vi "Install Package via Custom System Exec.vi"(8 "error in":errorcluster, 9 "include recommended packages? (F)":bool, 10 "version":string, 11 "package name":string) -> (0 "error out":errorcluster, 2 "installed version":string, 3 "package name out":string)   [LabVIEW 2019]
doc: "Installs the specified package on this computer.\n\nNote: This VI will launch a Windows dialog asking for permission to run and requires the user to have admin rights.\n\nINPUT(s)\n<B>Package name</B>: Specifies the package to install.\n\n<B>Version</B>:\nIf the version input is left unwired and no version of the package is currently installed, this VI will install the latest version of the package available from the registered feeds on the computer.\nIf the version input is left unwired and any version of the package is currently installed, this VI will output an error.\n\nIf the version input is wired and a different version of the package is installed, this VI will upgrade or downgrade the package to the specified version.\nIf the version input is wired and the specified version of the package is already installed, this VI will output an error.\n\n<B>Include recommended packages</B>: Also install all recommended packages of the specified package.\n\nOUTPUT(s)\n<B>Package name</B>: Outputs the requested package to install.\n\n<B>Installed version</B>: Outputs the currently installed version of the specified package after this VI tries to install the package.\n\nNIPM API 3.2.1.9\nNational Instruments\nCopyright (c) 2020, National Instruments"
uses:
  <vilib>/National Instruments/NIPM API (Beta)/NIPM_API.lvlib
  <vilib>/National Instruments/NIPM API (Beta)/_support/Version Comparison Operator.ctl
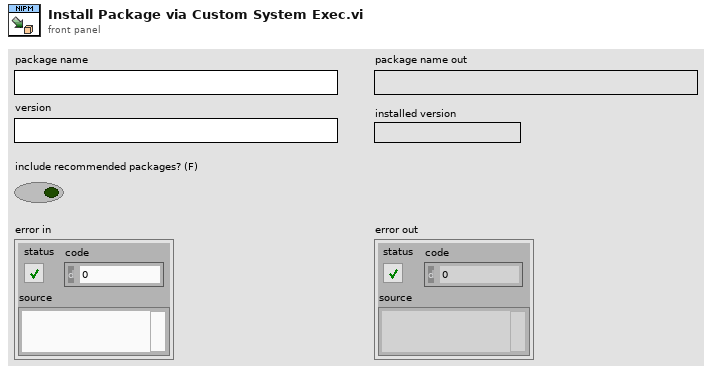
[diagram p1: front panel]
types:
  T1 = typedef "NIPM_API.lvlib/Version Comparison Operator.ctl" = enum16{">", ">=", "=", "!=", "<=", "<"}
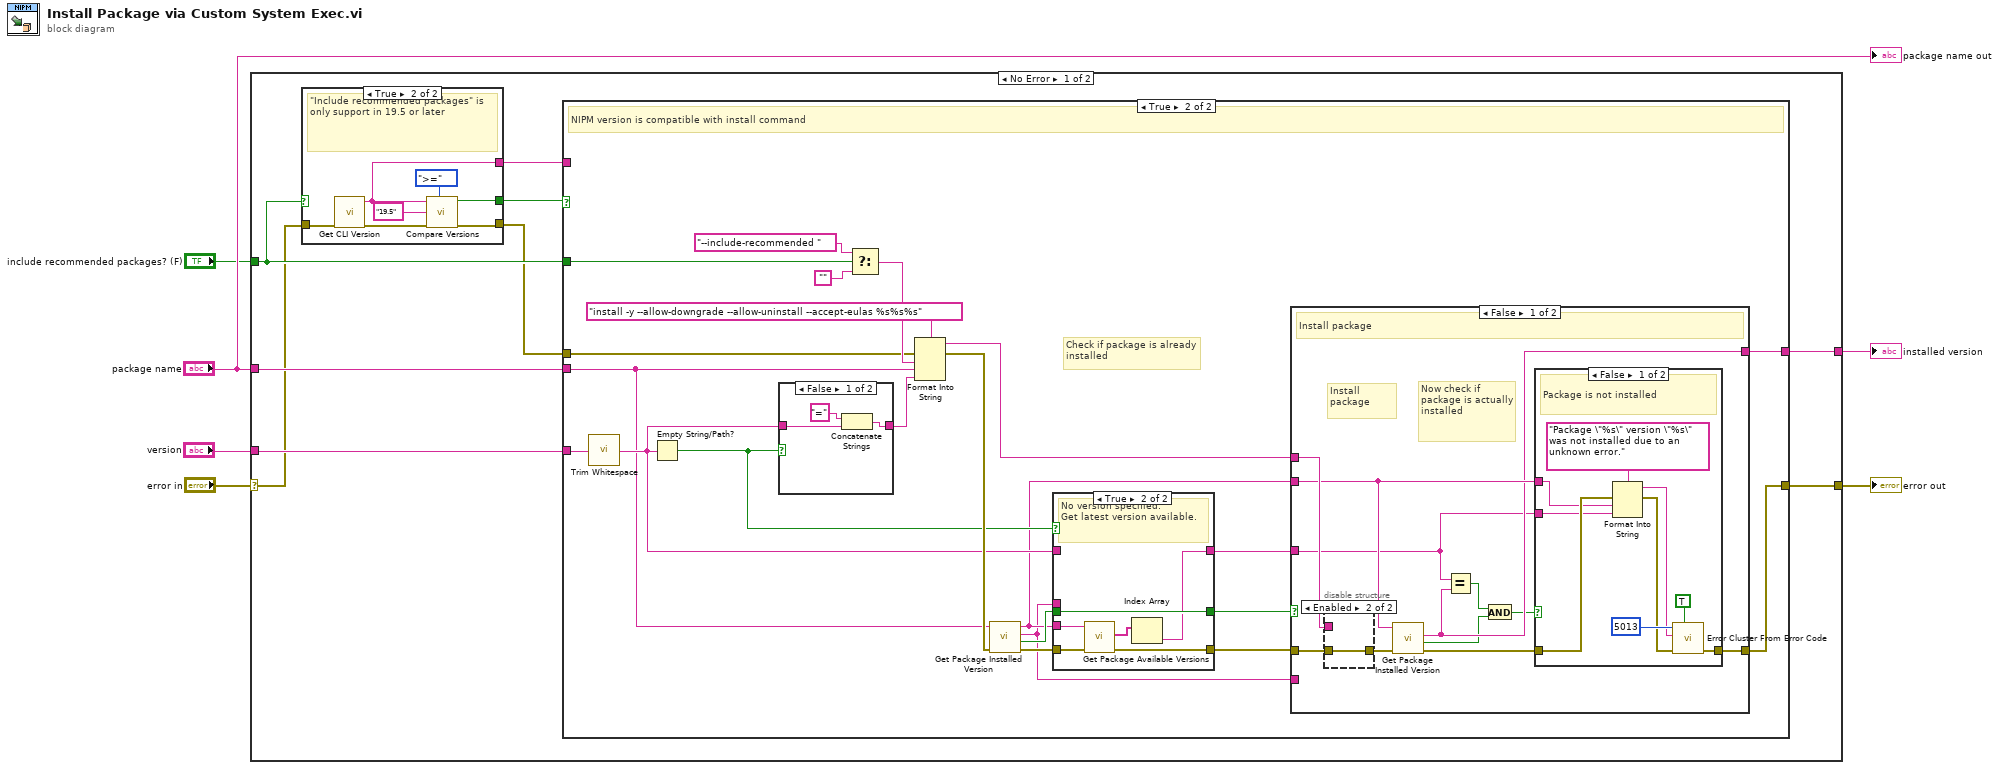
[diagram p0: block diagram]
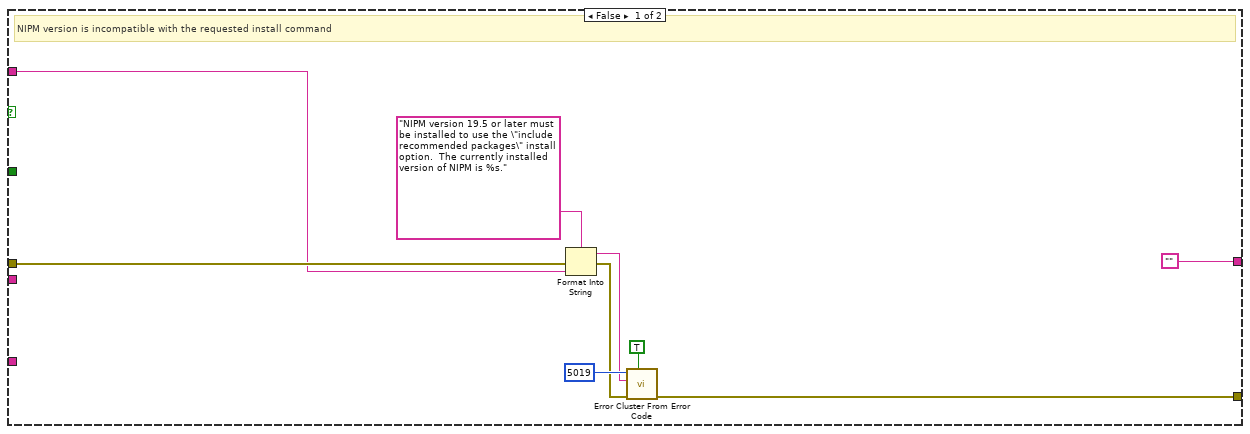
[diagram p2: hidden frame]
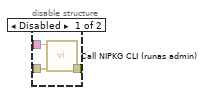
[diagram p3: hidden frame]
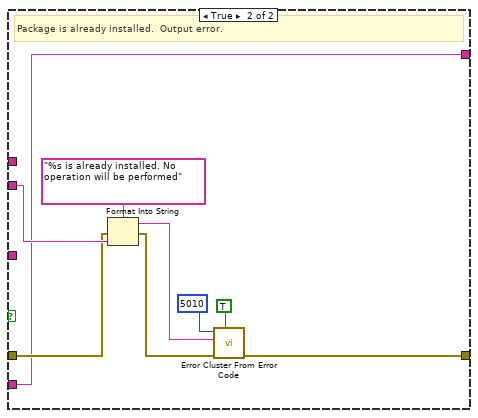
[diagram p5: hidden frame]
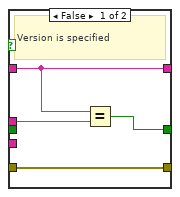
[diagram p6: hidden frame]
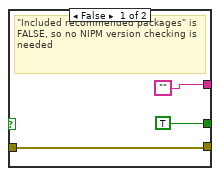
[diagram p8: hidden frame]
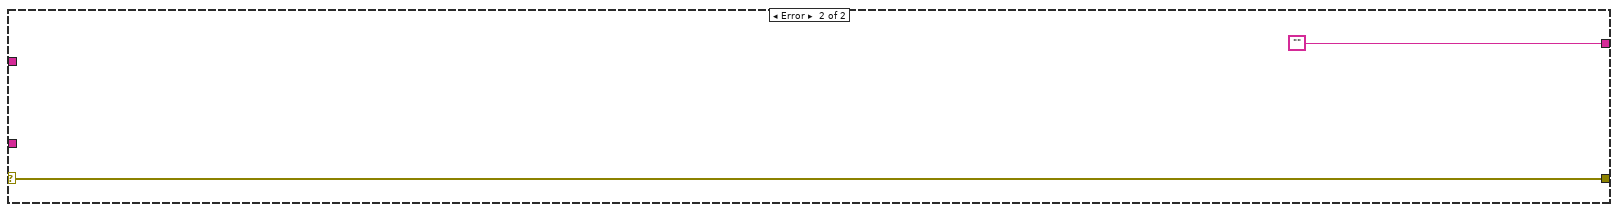
[diagram p9: hidden frame]
diagram:
  n1 = case shown="No Error" "error in" {
    selector: "error in" -> [w10 w106]
    tunnel: [w15 w106] -> w5
    tunnel: "package name" -> [w12 _]
    tunnel: "version" -> [w14 _]
    tunnel: [w13 "" ("standard output")] -> w2
    tunnel: "include recommended packages? (F)" -> [w11 _]
    frame No Error {
      n2 = case shown="True" w11 {
        tunnel: w10 -> [w97 w101]
        tunnel: [w97 w100] -> w9
        tunnel: [TRUE ("Satisfied?") w99] -> w8
        tunnel: ["" w98] -> w7
        frame False {
          # "\"Included recommended packages\" is FALSE, so no NIPM version checking is needed"
        }
        frame True {
          # "\"Include recommended packages\" is only support in 19.5 or later"
          n3 = call <vilib>:"Get CLI Version.vi"("error in"=w101) -> ("error out"=w102:errorcluster, "full version string"=w98:string)  [unwired: 9 in]
          n4 = call <vilib>:"Compare Versions.vi"("operator"=Version_Comparison_Operator.">=", "error in"=w102, "version y"="19.5", "version x"=w98) -> ("error out"=w100:errorcluster, "Satisfied?"=w99:bool)  [unwired: 6 in]
        }
      }
      n5 = case shown="True" w8 {
        tunnel: [w18 w42] -> w15
        tunnel: w14 -> [_ w40]
        tunnel: ["" w38] -> w13
        tunnel: w12 -> [_ w28]
        tunnel: w11 -> [_ w26]
        tunnel: w9 -> [w19 w25]
        tunnel: w7 -> [w16 _]
        frame False {
          # "NIPM version is incompatible with the requested install command"
          n6 = Format Into String(format string="NIPM version 19.5 or later must be installed to use the \"include recommended packages\" install option.  The currently installed version of NIPM is %s.", error in=w19, w16) -> (resulting string=w20:string, error out=w21:errorcluster)  [unwired: 1 in]
          n7 = call <vilib>:"Error Cluster From Error Code.vi"("show call chain? (False)"=TRUE, "error in (no error)"=w21, "error message (\"\")"=w20, "error code (0)"=5019) -> ("error out"=w18:errorcluster)  [unwired: 5 in]
        }
        frame True {
          # "Check if package is already installed"
          # "NIPM version is compatible with install command"
          n8 = call <vilib>:"Trim Whitespace.vi"("string"=w40) -> ("trimmed string"=w39:string)  [unwired: 1 in]
          n9 = Empty String/Path?(string/path=w39) -> (empty?=w41:bool)
          n10 = case shown="False" w41 {
            tunnel: w39 -> [w93 w94]
            tunnel: [w91 w94] -> w45
            frame False {
              n11 = Concatenate Strings("=" ("string"), w93) -> (w91:string)
            }
            frame True {
            }
          }
          n12 = Select(t="--include-recommended ", s=w26, f="") -> (s? t:f=w27:string)
          n13 = Format Into String(format string="install -y --allow-downgrade --allow-uninstall --accept-eulas %s%s%s", error in=w25, w27, w28, w45) -> (resulting string=w43:string, error out=w44:errorcluster)  [unwired: 1 in]
          n14 = call <vilib>:"Get Package Installed Version.vi"("error in"=w44, "package name"=w28) -> ("error out"=w34:errorcluster, "installed?"=w37:bool, "installed version"=w31:string, "package name out"=w32:string)  [unwired: 6 in]
          n15 = case shown="True" w41 {
            tunnel: w37 -> [_ w90]
            tunnel: w31 -> [w84 _]
            tunnel: w39 -> [w82 _]
            tunnel: [w83 w90] -> w36
            tunnel: [w82 w87] -> w35
            tunnel: w34 -> [w81 w89]
            tunnel: [w81 w86] -> w33
            tunnel: w32 -> [_ w85]
            frame False {
              # "Version is specified"
              n16 = Equal?(x=w82, y=w84) -> (x = y?=w83:bool)
            }
            frame True {
              # "No version specified.\nGet latest version available."
              n17 = call <vilib>:"Get Package Available Versions.vi"("error in"=w89, "package name"=w85) -> ("error out"=w86:errorcluster, "versions"=w88:string[])  [unwired: 7 in, 1 out]
              n18 = Index Array(array=w88) -> (element=w87:string)  [unwired: 1 in]
            }
          }
          n19 = case shown="False" w36 {
            tunnel: w43 -> [w57 _]
            tunnel: [w53 w73] -> w42
            tunnel: w33 -> [w56 w75]
            tunnel: w32 -> [w52 w77]
            tunnel: w35 -> [w50 _]
            tunnel: [w51 w72] -> w38
            tunnel: w31 -> [_ w72]
            frame False {
              # "Install package"
              # "Now check if package is actually installed"
              # "Install package"
              n20 = disable-structure shown="Enabled" {
                disable-tunnel: w57 -> [w60 _]
                disable-tunnel: w56 -> [w59 w61]
                disable-tunnel: [w58 w61] -> w55
                frame Disabled {
                  n21 = call <vilib>:"Call NIPKG CLI (runas admin).vi"("error in (no error)"=w59, "command"=w60) -> ("error out"=w58:errorcluster)  [unwired: 9 in]
                }
                frame Enabled {
                }
              }
              n22 = call <vilib>:"Get Package Installed Version.vi"("error in"=w55, "package name"=w52) -> ("error out"=w54:errorcluster, "installed?"=w47:bool, "installed version"=w51:string)  [unwired: 6 in, 1 out]
              n23 = Equal?(x=w50, y=w51) -> (x = y?=w49:bool)
              n24 = And(x=w49, y=w47) -> (x .and. y?=w48:bool)
              n25 = case shown="False" w48 {
                tunnel: w54 -> [w65 w71]
                tunnel: [w68 w71] -> w53
                tunnel: w52 -> [w64 _]
                tunnel: w50 -> [w62 _]
                frame False {
                  # "Package is not installed"
                  n26 = Format Into String(format string="Package \"%s\" version \"%s\" was not installed due to an unknown error.", error in=w65, w64, w62) -> (resulting string=w63:string, error out=w66:errorcluster)  [unwired: 1 in]
                  n27 = call <vilib>:"Error Cluster From Error Code.vi"("show call chain? (False)"=TRUE, "error in (no error)"=w66, "error message (\"\")"=w63, "error code (0)"=5013) -> ("error out"=w68:errorcluster)  [unwired: 5 in]
                }
                frame True {
                  # "Package has installed successfully."
                }
              }
            }
            frame True {
              # "Package is already installed.  Output error."
              n28 = Format Into String(format string="%s is already installed. No operation will be performed", error in=w75, w77) -> (resulting string=w76:string, error out=w74:errorcluster)  [unwired: 1 in]
              n29 = call <vilib>:"Error Cluster From Error Code.vi"("show call chain? (False)"=TRUE, "error in (no error)"=w74, "error message (\"\")"=w76, "error code (0)"=5010) -> ("error out"=w73:errorcluster)  [unwired: 5 in]
            }
          }
        }
      }
    }
    frame Error {
    }
  }
  "error out" <- w5
  "installed version" <- w2
  "package name out" <- "package name"
